vi "Ramprate Conversion Constant.vi"() -> (8 "ramp rate conversion constant":dbl)   [LabVIEW 2024, in "devicePowerSequencerCoreLogic.lvlib"]
uses:
  devicePowerSequencerCoreLogic.lvlib
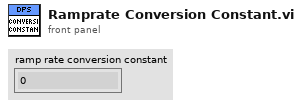
[diagram p1: front panel]
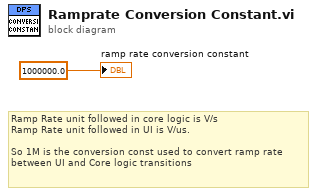
[diagram p0: block diagram]
diagram:
  # "Ramp Rate unit followed in core logic is V/s\nRamp Rate unit followed in UI is V/us.\n\nSo 1M is the conversion const used to convert ramp rate\nbetween UI and Core logic transitions"
  "ramp rate conversion constant" <- 1000000.0 ("y")
